vi "Single Shot Application.vi"() -> ()   [LabVIEW 2012]
doc: "This sample project is built upon the standard state machine template and shows how you could create an application that acquires, analyzes, and presents data. It includes functionality for presenting configuration dialogs, preserving settings between executions, loading and saving data, as well as exporting graph images and text files.\n\nIt is most appropriate for data that is acquired instantly as it does not allow for screen updates mid acquisition nor does it allow for continuous streaming to disk."
uses:
  controls/Acquire_Type.ctl
  controls/MDOData.ctl
  controls/MDOUI References.ctl
  controls/MDOGraph Data.ctl
  <vilib>/Utility/miscctls.llb/LVAnnotationListTypeDef.ctl
  <vilib>/Utility/miscctls.llb/LVCursorListTypeDef.ctl
  controls/MDOUser Specified Data.ctl
  controls/MDOHW Configuration.ctl
  controls/MDONew Data Behavior.ctl
  controls/Coeff.ctl
  controls/MDOState.ctl
  <vilib>/Analysis/baseanly.llb/Mean (DBL).vi
  <vilib>/Analysis/NI_AALBase.lvlib
panel:
  in  "Calibrate":bool
  out "Acquire Type":T1=enum."Continues"
  in  "Cancel":bool
  in  "Settings":bool
  in  "Snapshot":bool
  in  "Analyze":bool
  in  "Clear":bool
  in  "Stop":bool
  in  "Acquire":bool
  in  "Export":bool
  in  "Save Data":bool
  in  "Load Data":bool
  out "Mixed Signal Graph":cluster{waveform(dbl)[], waveform(dbl)[]}(graph)
  out "Status Bar":string
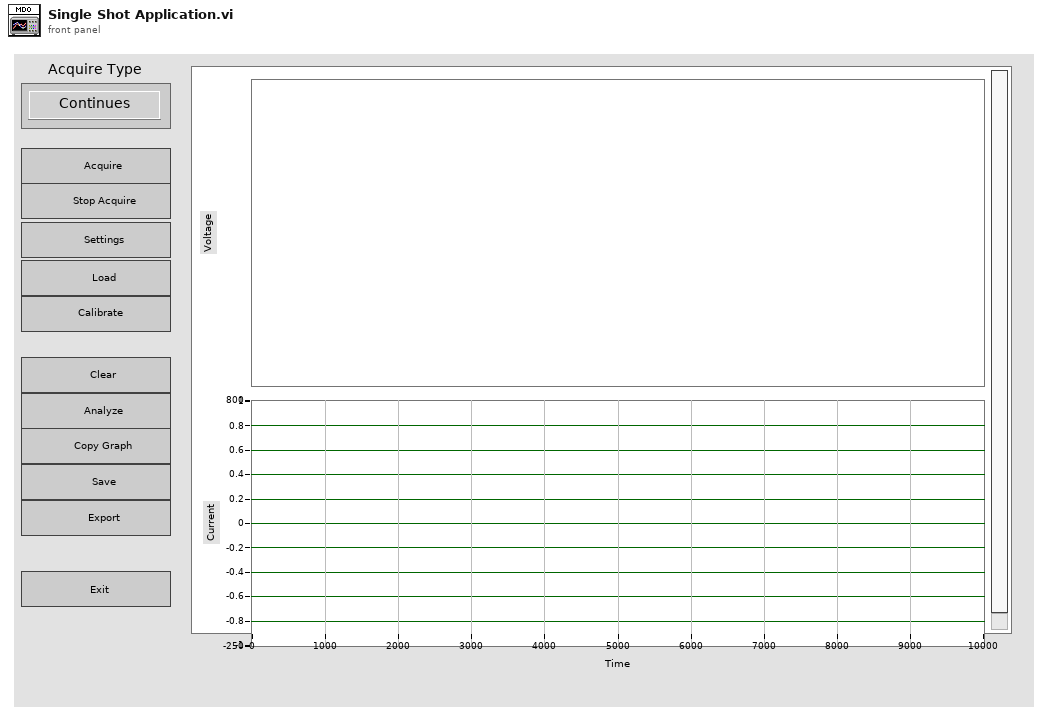
[diagram p1: front panel]
types:
  T1 = typedef "Acquire_Type.ctl" = enum16{"Triggered", "Continues"}
  T2 = typedef "MDOState.ctl" = enum16{"Wait for Event", "Initialize", "Update UI", "Configure", "Single Acquire", "Stop Contin Acquire", "Load Data", "Save Data", "Clear Data", "Export Data", "Analyze", "Copy Graph", "Calibrate", "Stop", "Run Contin Asquire", "Monitor Contin Asquire"}
  T3 = typedef "MDOData.ctl" = cluster{"UI References":T4, "Graph Data":T5, "User Specified":T8, "Coeff":T11}
  T4 = typedef "MDOUI References.ctl" = cluster{"Stop Ref":refnum<vi>, "Save Ref":refnum<vi>, "Open Ref":refnum<vi>, "Export Ref":refnum<vi>, "Acquire Ref":refnum<vi>, "Configure Ref":refnum<vi>, "Clear Ref":refnum<vi>, "Analyze Ref":refnum<vi>, "Status Ref":refnum<vi>, "Snapshot Ref":refnum<vi>, "Cancel":refnum<vi>, "Graph Ref":refnum<vi>}
  T5 = typedef "MDOGraph Data.ctl" = cluster{"Voltage Data":waveform(dbl)[], "Annotation List":T6, "Cursor List":T7, "Voltage Analysis Data":waveform(dbl)[], "Current Data":waveform(dbl)[], "Current Analysis Data":waveform(dbl)[]}
  T6 = typedef "LVAnnotationListTypeDef.ctl" = cluster{"Name":string, "Color":u32, "Style":u8, "Point Style":u8, "Name Visible":bool, "Allow Drag":bool, "Annotation Mode":u32, "Plot":i32, "Index":i32, "Position":cluster{"X":dbl, "Y":dbl}, "X Scale":u32, "Y Scale":u32, "Show Arrow":bool, "Lock Name":bool, "Plot Area":i32, "Label Offset":cluster{"X":dbl, "Y":dbl}}[]
  T7 = typedef "LVCursorListTypeDef.ctl" = cluster{"Name":string, "Color":u32, "Style":u8, "Point Style":u8, "Name Visible":bool, "Allow Drag":bool, "Cursor Mode":u32, "Plot":i32, "Index":i32, "Position":cluster{"X":dbl, "Y":dbl}, "X Scale":u32, "Y Scale":u32, "Watch Plots":i32[], "Watch All Plots":bool, "Plot Area":i32, "Label Offset":cluster{"X":dbl, "Y":dbl}}[]
  T8 = typedef "MDOUser Specified Data.ctl" = cluster{"Hardware Configuration":T9, "New Data Behavior":T10, "Acquire Type":T1, "Data_save_directory":path}
  T9 = typedef "MDOHW Configuration.ctl" = cluster{"SyncMode":u32, "Current_FIR_filter":bool}
  T10 = typedef "MDONew Data Behavior.ctl" = enum16{"Replace", "Overlay", "Append"}
  T11 = typedef "Coeff.ctl" = cluster{"Coeff_U":dbl, "Offset_U":dbl, "Coeff_I":dbl, "Offset_I":dbl}
  T12 = enum32{"invalid app kind", "Development System", "Run Time System", "Student Edition", "Embedded LabVIEW", "Evaluation", "Custom"}
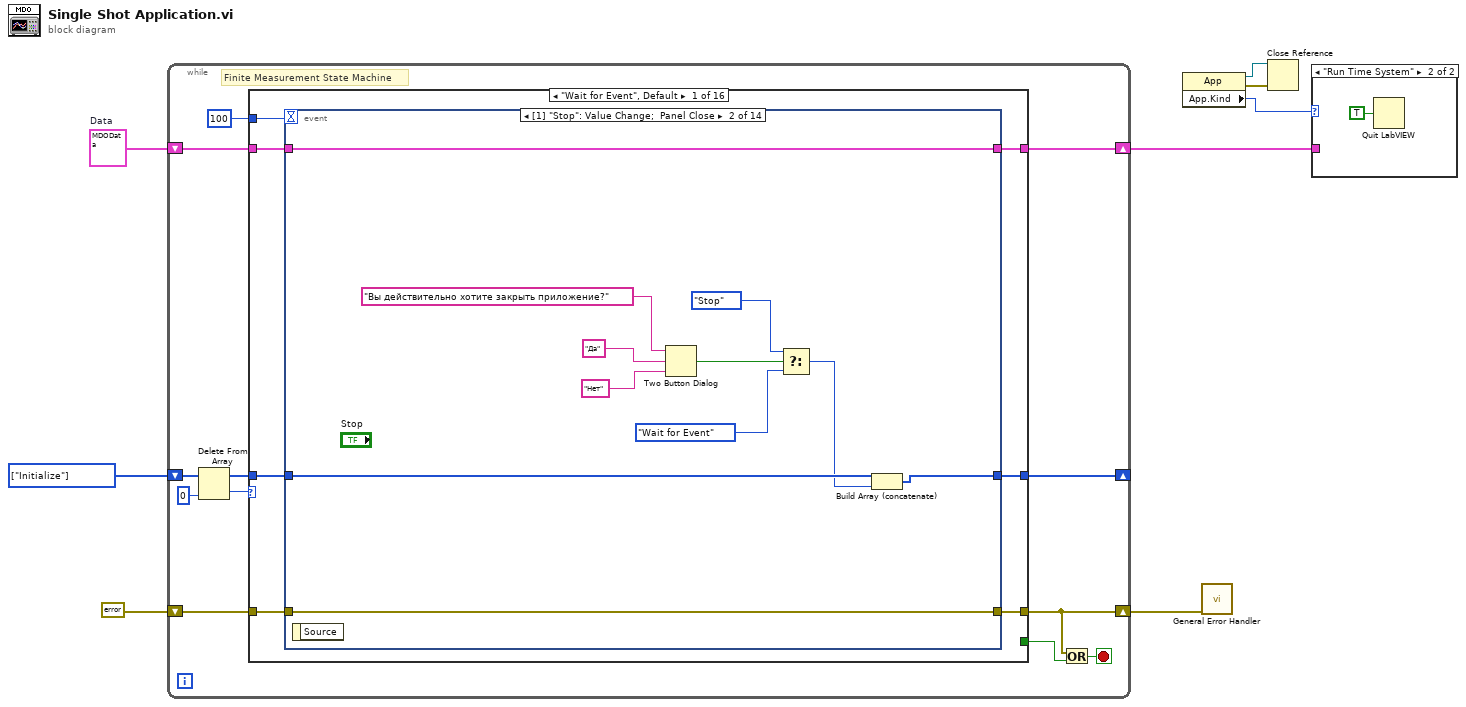
[diagram p0: block diagram]
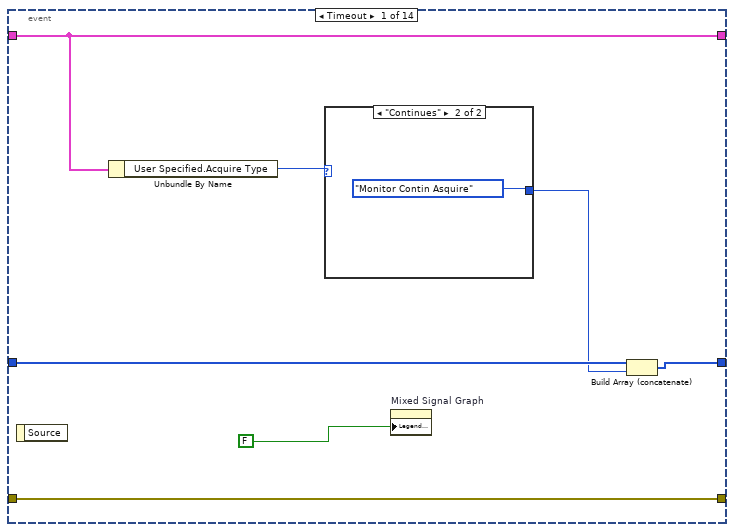
[diagram p3: hidden frame]
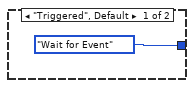
[diagram p4: hidden frame]
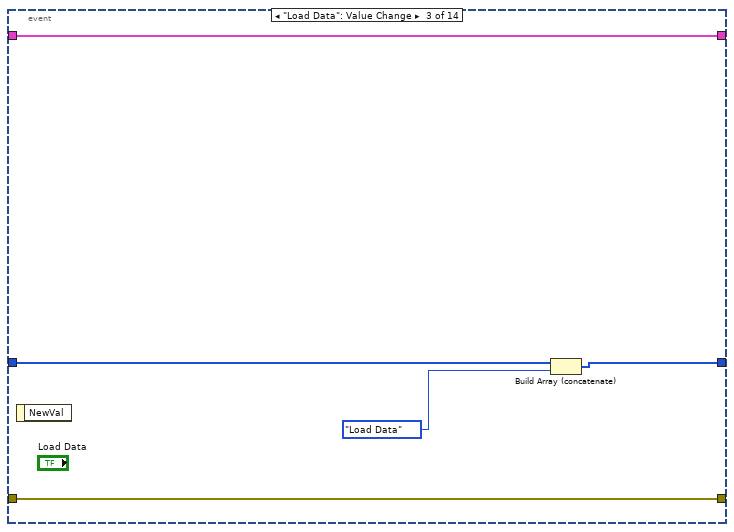
[diagram p5: hidden frame]
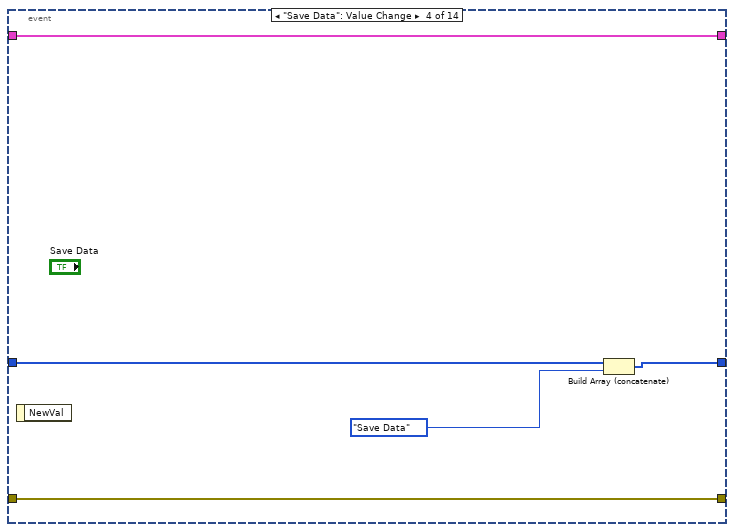
[diagram p6: hidden frame]
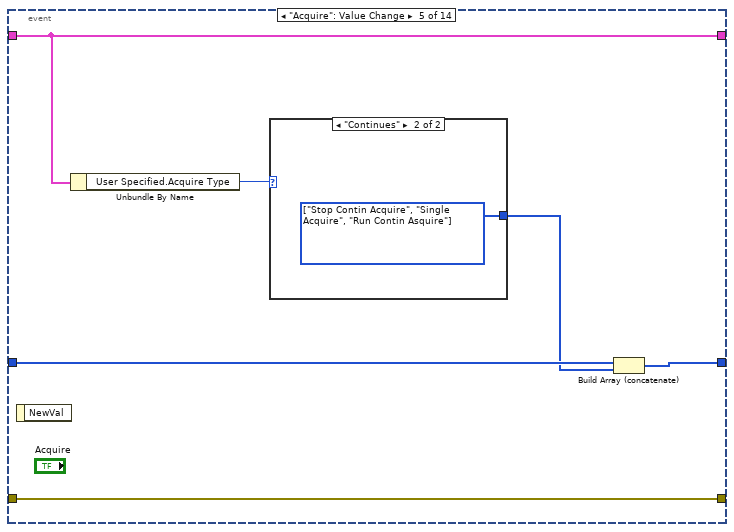
[diagram p7: hidden frame]
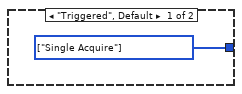
[diagram p8: hidden frame]
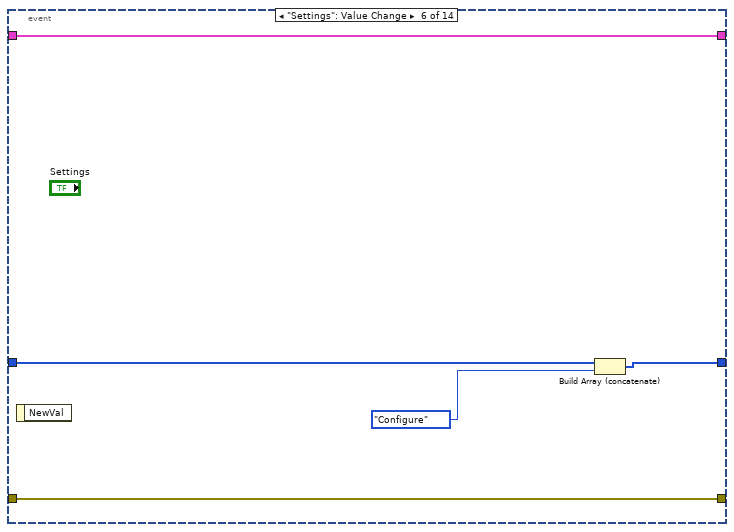
[diagram p9: hidden frame]
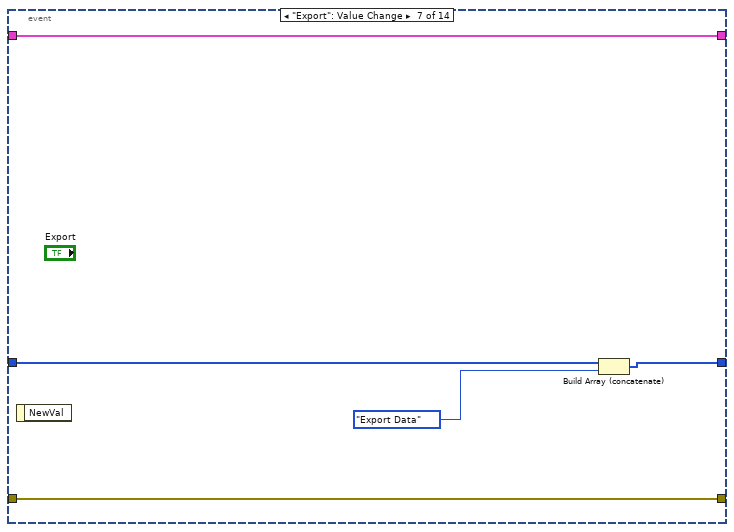
[diagram p10: hidden frame]
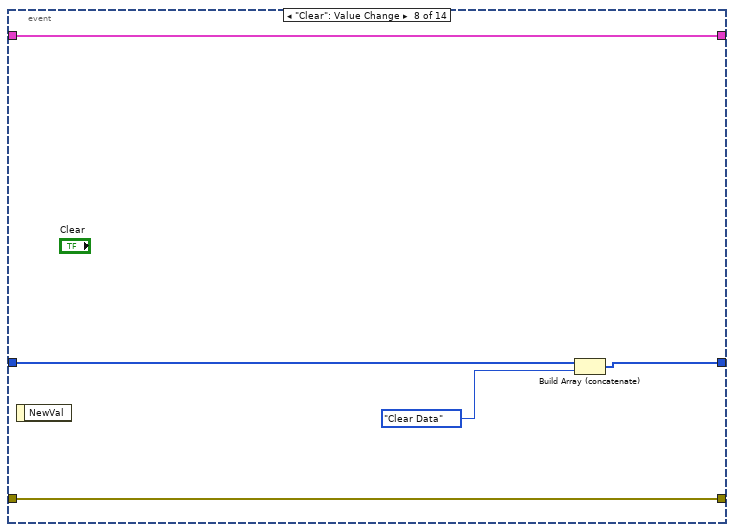
[diagram p11: hidden frame]
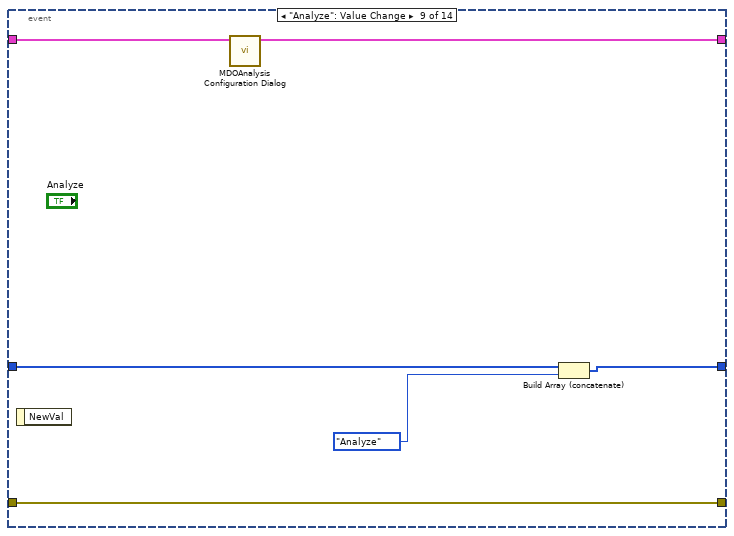
[diagram p12: hidden frame]
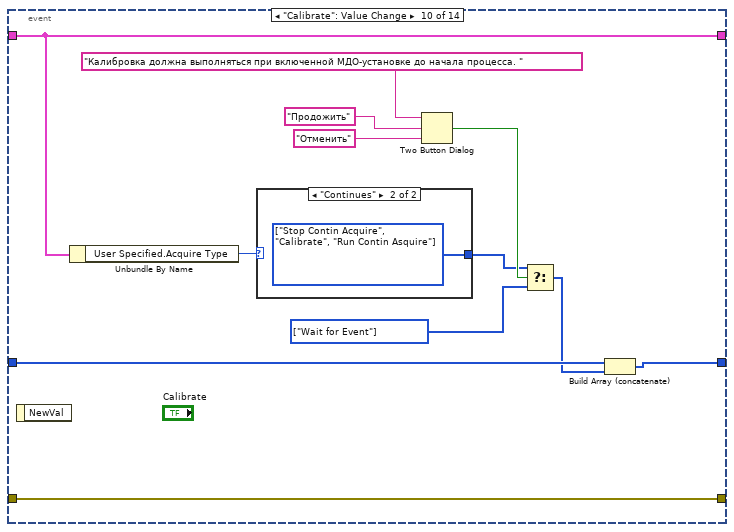
[diagram p13: hidden frame]
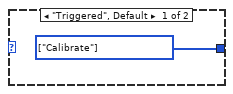
[diagram p14: hidden frame]
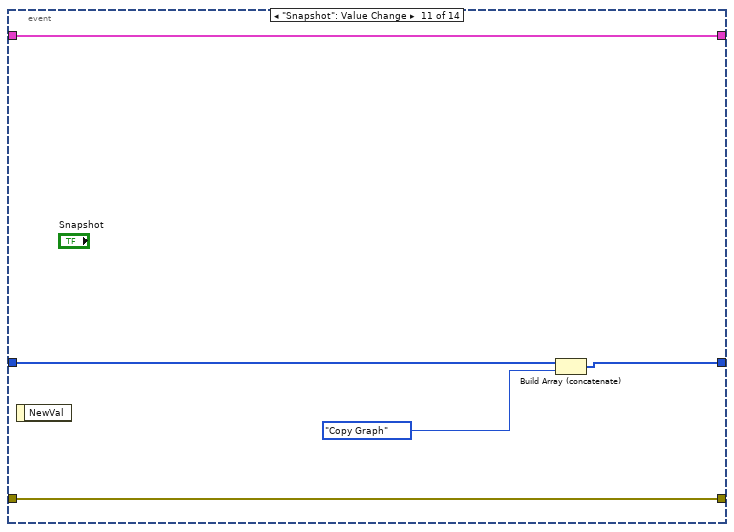
[diagram p15: hidden frame]
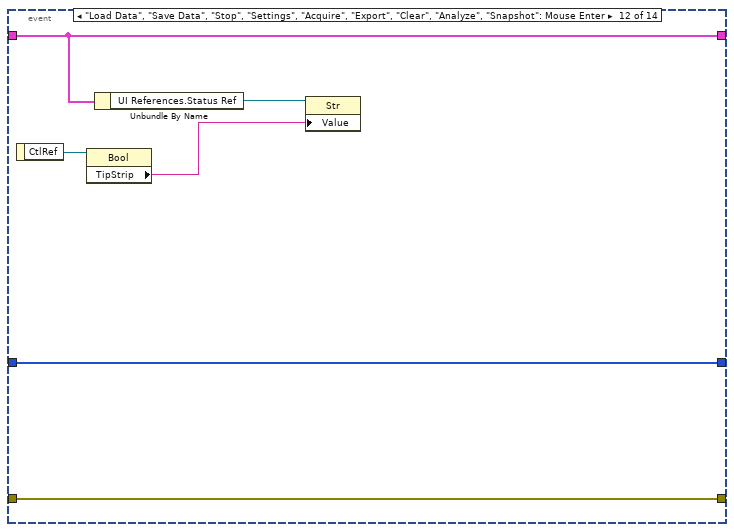
[diagram p16: hidden frame]
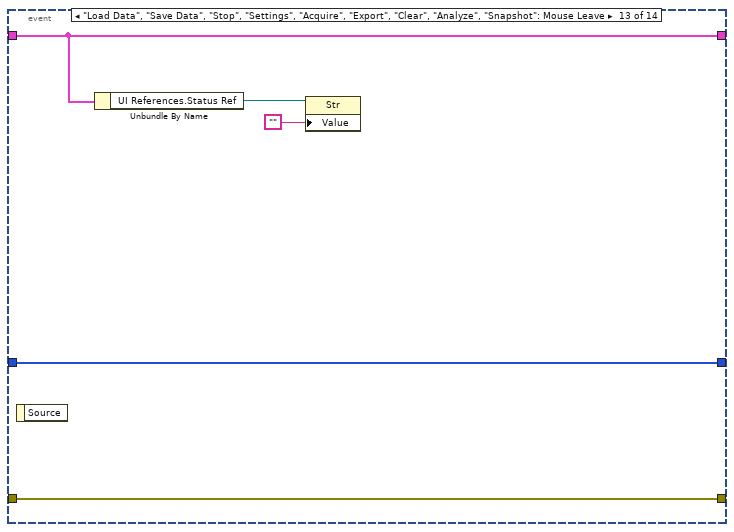
[diagram p17: hidden frame]
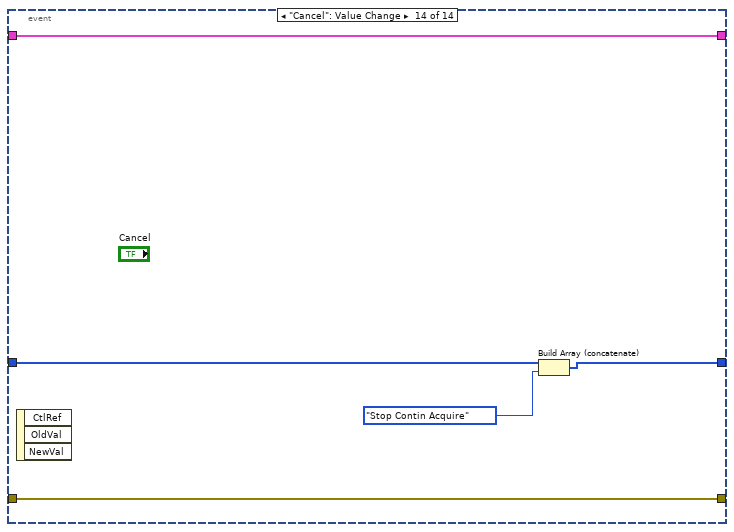
[diagram p18: hidden frame]
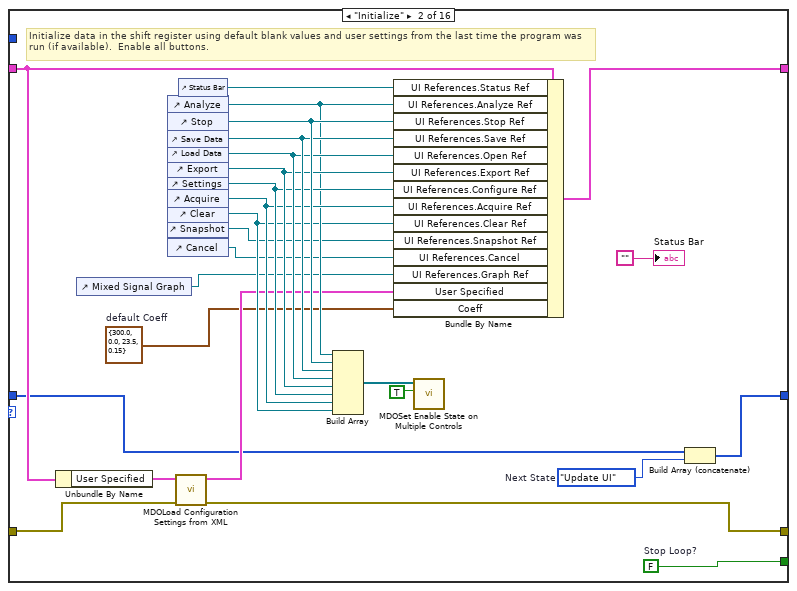
[diagram p19: hidden frame]
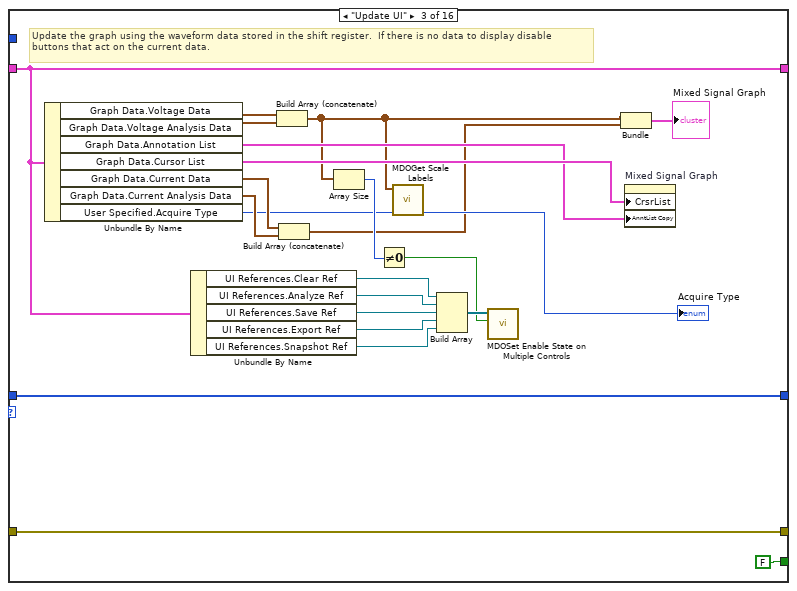
[diagram p20: hidden frame]
diagram:
  w1 = T2[] [enum."Initialize"] items=["Wait for Event", "Initialize", "Update UI", "Configure", "Single Acquire", "Stop Contin Acquire", "Load Data", "Save Data", "Clear Data", "Export Data", "Analyze", "Copy Graph", "Calibrate", "Stop", "Run Contin Asquire", "Monitor Contin Asquire"]
  w2 = T3 {"UI References"={"Stop Ref"=refnum, "Save Ref"=refnum, "Open Ref"=refnum, "Export Ref"=refnum, "Acquire Ref"=refnum, "Configure Ref"=refnum, "Clear Ref"=refnum, "Analyze Ref"=refnum, "Status Ref"=refnum, "Snapshot Ref"=refnum, "Cancel"=refnum, "Graph Ref"=refnum}, "Graph Data"={"Voltage Data"=[], "Annotation List"=[], "Cursor List"=[], "Voltage Analysis Data"=[], "Current Data"=[], "Current Analysis Data"=[]}, "User Specified"={"Hardware Configuration"={"SyncMode"=0, "Current_FIR_filter"=FALSE}, "New Data Behavior"=enum."Replace", "Acquire Type"=enum."Triggered", "Data_save_directory"=path ""}, "Coeff"={"Coeff_U"=0.0, "Offset_U"=0.0, "Coeff_I"=0.0, "Offset_I"=0.0}}  # Data
  n1 = while {
    shift-right: [w9] -> _
    shift-left: w1 -> [w14]
    shift-right: [w19] -> w3
    shift-left: w2 -> [w20]
    shift-right: [w15] -> w7
    shift-left: errorcluster {"status"=FALSE, "code"=0, "source"=""} ("error constant") -> [w18]
    stop <- w16 stop-if-true
    # "Finite Measurement State Machine"
    n2 = Delete From Array(array=w14, index=0) -> (deleted portion=w12:T2, array with subset deleted=w11:T2[])  [unwired: 1 in]
    n3 = case shown="\"Wait for Event\", Default" w12 {
      tunnel: [_ w147 FALSE ("Stop Loop?") FALSE ("Stop Loop?") FALSE ("Stop Loop?") FALSE ("Stop Loop?") FALSE ("Stop Loop?") FALSE ("Stop Loop?") FALSE ("Stop Loop?") FALSE ("Stop Loop?") FALSE ("Stop Loop?") FALSE ("Stop Loop?") FALSE ("Stop Loop?") w334 FALSE ("Stop Loop?") FALSE ("Stop Loop?")] -> w17
      tunnel: w20 -> [w27 w138 w168 w181 w195 w228 w244 w263 w276 w283 w297 w303 w310 w332 w346 w370]
      tunnel: [w26 w146 w168 w180 w194 w228 w239 w263 w275 w283 w297 w303 w309 w332 w346 w369] -> w19
      tunnel: w18 -> [w25 w125 w169 w179 w191 w226 w243 w265 w277 w286 w292 w302 w308 w329 w350 _]
      tunnel: [w24 w126 w169 w178 w192 w225 w242 w261 w277 w280 w291 w301 w308 w328 w350 w368] -> w15
      tunnel: w11 -> [w22 w124 w148 w172 w185 w221 w231 w255 w272 w278 w295 w299 w306 w327 w335 w353]
      tunnel: 100 -> [w23 _ _ _ _ _ _ _ _ _ _ _ _ _ _ _]
      tunnel: [w21 w122 w148 w170 w183 w219 w229 w255 w270 w278 w293 w299 w304 w325 w335 w351] -> w9
      frame "Wait for Event", Default {
        n4 = event shown="[1] \"Stop\": Value Change;  Panel Close" {
          selector: _ -> [_ _ _ _ _ _ _ _ _ _ _ _ _ _]
          dyn-events: _ -> [_ _ _ _ _ _ _ _ _ _ _ _ _ _]
          timeout: w23 -> [_ _ _ _ _ _ _ _ _ _ _ _ _ _]
          tunnel: w27 -> [w33 w47 w52 w57 w62 w70 w75 w80 w85 w91 w105 w109 w115 w121]
          tunnel: [w33 w47 w52 w57 w62 w70 w75 w80 w84 w91 w105 w109 w115 w121] -> w26
          tunnel: w25 -> [w34 w46 w51 w56 w63 w69 w74 w79 w86 w98 w104 w111 w116 w120]
          tunnel: [w34 w46 w51 w56 w63 w69 w74 w79 w86 w98 w104 w111 w116 w120] -> w24
          tunnel: w22 -> [w31 w45 w50 w55 w60 w68 w73 w78 w83 w93 w103 w106 w112 w119]
          tunnel: [w30 w44 w48 w53 w59 w66 w71 w76 w81 w92 w101 w106 w112 w117] -> w21
          event Timeout {
            n5 = event-data() -> ()  [unwired: 1 in, 1 out]
            n6 = Unbundle By Name(w33) -> ("User Specified.Acquire Type"=w32:T1)
            n7 = case shown="\"Continues\"" w32 {
              tunnel: [MDOState."Wait for Event" ("Next State") MDOState."Monitor Contin Asquire" ("Next State")] -> w29
              frame "Triggered", Default {
              }
              frame "Continues" {
              }
            }
            n8 = property on="Mixed Signal Graph" class="MixedGraph (strict)"("Legend Visible"=FALSE ("Boolean")) -> ()  [unwired: 2 in, 2 out]
            n9 = Build Array (concatenate)(w31, w29) -> (w30:T2[])
          }
          event "Stop": Value Change; Panel Close {
            n10 = event-data() -> ()  [unwired: 1 in, 1 out]
            n11 = Two Button Dialog(message="Вы действительно хотите закрыть приложение?", 1:"Нет" ("F button name (\"Cancel\")"), 2:"Да" ("T button name (\"OK\")")) -> (T button?=w40:bool)
            n12 = Select(t=MDOState."Stop" ("Next State"), s=w40, f=MDOState."Wait for Event" ("Next State")) -> (s? t:f=w37:T2)
            n13 = Build Array (concatenate)(w45, w37) -> (w44:T2[])
          }
          event "Load Data": Value Change {
            n14 = event-data() -> ()  [unwired: 1 in, 1 out]
            n15 = Build Array (concatenate)(w50, MDOState."Load Data" ("Next State")) -> (w48:T2[])
          }
          event "Save Data": Value Change {
            n16 = event-data() -> ()  [unwired: 1 in, 1 out]
            n17 = Build Array (concatenate)(w55, MDOState."Save Data" ("Next State")) -> (w53:T2[])
          }
          event "Acquire": Value Change {
            n18 = event-data() -> ()  [unwired: 1 in, 1 out]
            n19 = Unbundle By Name(w62) -> ("User Specified.Acquire Type"=w61:T1)
            n20 = case shown="\"Continues\"" w61 {
              tunnel: [w64 w65] -> w58
              frame "Triggered", Default {
                w64 = T2[] [enum."Single Acquire"] items=["Wait for Event", "Initialize", "Update UI", "Configure", "Single Acquire", "Stop Contin Acquire", "Load Data", "Save Data", "Clear Data", "Export Data", "Analyze", "Copy Graph", "Calibrate", "Stop", "Run Contin Asquire", "Monitor Contin Asquire"] ("array")
              }
              frame "Continues" {
                w65 = T2[] [enum."Stop Contin Acquire", enum."Single Acquire", enum."Run Contin Asquire"] items=["Wait for Event", "Initialize", "Update UI", "Configure", "Single Acquire", "Stop Contin Acquire", "Load Data", "Save Data", "Clear Data", "Export Data", "Analyze", "Copy Graph", "Calibrate", "Stop", "Run Contin Asquire", "Monitor Contin Asquire"] ("array")
              }
            }
            n21 = Build Array (concatenate)(w60, w58) -> (w59:T2[])
          }
          event "Settings": Value Change {
            n22 = event-data() -> ()  [unwired: 1 in, 1 out]
            n23 = Build Array (concatenate)(w68, MDOState."Configure" ("Next State")) -> (w66:T2[])
          }
          event "Export": Value Change {
            n24 = event-data() -> ()  [unwired: 1 in, 1 out]
            n25 = Build Array (concatenate)(w73, MDOState."Export Data" ("Next State")) -> (w71:T2[])
          }
          event "Clear": Value Change {
            n26 = event-data() -> ()  [unwired: 1 in, 1 out]
            n27 = Build Array (concatenate)(w78, MDOState."Clear Data" ("Next State")) -> (w76:T2[])
          }
          event "Analyze": Value Change {
            n28 = event-data() -> ()  [unwired: 1 in, 1 out]
            n29 = call "MDOAnalysis Configuration Dialog.vi"("Data in"=w85) -> ("Data out"=w84:T3)  [unwired: 10 in]
            n30 = Build Array (concatenate)(w83, MDOState."Analyze" ("Next State")) -> (w81:T2[])
          }
          event "Calibrate": Value Change {
            w90 = T2[] [enum."Wait for Event"] items=["Wait for Event", "Initialize", "Update UI", "Configure", "Single Acquire", "Stop Contin Acquire", "Load Data", "Save Data", "Clear Data", "Export Data", "Analyze", "Copy Graph", "Calibrate", "Stop", "Run Contin Asquire", "Monitor Contin Asquire"] ("array")
            n31 = event-data() -> ()  [unwired: 1 in, 1 out]
            n32 = Unbundle By Name(w91) -> ("User Specified.Acquire Type"=w89:T1)
            n33 = case shown="\"Continues\"" w89 {
              tunnel: [w99 w100] -> w88
              frame "Triggered", Default {
                w99 = T2[] [enum."Calibrate"] items=["Wait for Event", "Initialize", "Update UI", "Configure", "Single Acquire", "Stop Contin Acquire", "Load Data", "Save Data", "Clear Data", "Export Data", "Analyze", "Copy Graph", "Calibrate", "Stop", "Run Contin Asquire", "Monitor Contin Asquire"] ("array")
              }
              frame "Continues" {
                w100 = T2[] [enum."Stop Contin Acquire", enum."Calibrate", enum."Run Contin Asquire"] items=["Wait for Event", "Initialize", "Update UI", "Configure", "Single Acquire", "Stop Contin Acquire", "Load Data", "Save Data", "Clear Data", "Export Data", "Analyze", "Copy Graph", "Calibrate", "Stop", "Run Contin Asquire", "Monitor Contin Asquire"] ("array")
              }
            }
            n34 = Two Button Dialog(message="Калибровка должна выполняться при включенной МДО-установке до начала процесса. ", 1:"Отменить" ("F button name (\"Cancel\")"), 2:"Продожить" ("T button name (\"OK\")")) -> (T button?=w94:bool)
            n35 = Select(t=w88, s=w94, f=w90) -> (s? t:f=w87:T2[])
            n36 = Build Array (concatenate)(w93, w87) -> (w92:T2[])
          }
          event "Snapshot": Value Change {
            n37 = event-data() -> ()  [unwired: 1 in, 1 out]
            n38 = Build Array (concatenate)(w103, MDOState."Copy Graph" ("Next State")) -> (w101:T2[])
          }
          event "Load Data", "Save Data", "Stop", "Settings", "Acquire", "Export", "Clear", "Analyze", "Snapshot": Mouse Enter {
            n39 = event-data() -> ("CtlRef"=w110:refnum<vi>)  [unwired: 1 in]
            n40 = property class="Bool"(reference=w110) -> ("TipStrip"=w107:string)  [unwired: 1 in, 2 out]
            n41 = Unbundle By Name(w109) -> ("UI References.Status Ref"=w108:refnum<vi>)
            n42 = property class="Str"(reference=w108, "Value"=w107) -> ()  [unwired: 1 in, 2 out]
          }
          event "Load Data", "Save Data", "Stop", "Settings", "Acquire", "Export", "Clear", "Analyze", "Snapshot": Mouse Leave {
            n43 = event-data() -> ()  [unwired: 1 in, 1 out]
            n44 = Unbundle By Name(w115) -> ("UI References.Status Ref"=w114:refnum<vi>)
            n45 = property class="Str"(reference=w114, "Value"="") -> ()  [unwired: 1 in, 2 out]
          }
          event "Cancel": Value Change {
            n46 = event-data() -> ()  [unwired: 1 in, 3 out]
            n47 = Build Array (concatenate)(w119, MDOState."Stop Contin Acquire" ("Initial State")) -> (w117:T2[])
          }
        }
      }
      frame "Initialize" {
        w127 = T11 {"Coeff_U"=300.0, "Offset_U"=0.0, "Coeff_I"=23.5, "Offset_I"=0.15}  # default Coeff
        w147 = FALSE  # Stop Loop?
        w123 = MDOState."Update UI"  # Next State
        # "Initialize data in the shift register using default blank values and user settings from the last time the program was run (if available).  Enable all buttons."
        n48 = Unbundle By Name(w138) -> ("User Specified"=w137:T8)
        n49 = control-ref of="Mixed Signal Graph"() -> (w128:refnum<vi>)
        n50 = control-ref of="Analyze"() -> (w136:refnum<vi>)
        n51 = control-ref of="Stop"() -> (w145:refnum<vi>)
        n52 = control-ref of="Save Data"() -> (w144:refnum<vi>)
        n53 = control-ref of="Load Data"() -> (w143:refnum<vi>)
        n54 = control-ref of="Export"() -> (w142:refnum<vi>)
        n55 = control-ref of="Settings"() -> (w141:refnum<vi>)
        n56 = control-ref of="Acquire"() -> (w140:refnum<vi>)
        n57 = control-ref of="Clear"() -> (w134:refnum<vi>)
        n58 = control-ref of="Snapshot"() -> (w131:refnum<vi>)
        n59 = control-ref of="Cancel"() -> (w129:refnum<vi>)
        n60 = call "MDOLoad Configuration Settings from XML.vi"("error in (no error)"=w125, "User Configuration in"=w137) -> ("error out"=w126:errorcluster, "User Configuration out"=w130:T8)  [unwired: 8 in]
        n61 = control-ref of="Status Bar"() -> (w135:refnum<vi>)
        n62 = Build Array(w136, w145, w144, w143, w142, w141, w140, w134) -> (w139:refnum<vi>[])
        n63 = Bundle By Name(cluster=w138, "UI References.Status Ref"=w135, "UI References.Analyze Ref"=w136, "UI References.Stop Ref"=w145, "UI References.Save Ref"=w144, "UI References.Open Ref"=w143, "UI References.Export Ref"=w142, "UI References.Configure Ref"=w141, "UI References.Acquire Ref"=w140, "UI References.Clear Ref"=w134, "UI References.Snapshot Ref"=w131, "UI References.Cancel"=w129, "UI References.Graph Ref"=w128, "User Specified"=w130, "Coeff"=w127) -> (w146:T3)
        n64 = call "MDOSet Enable State on Multiple Controls.vi"("Enable?"=TRUE, "Controls"=w139) -> ()  [unwired: 10 in]
        n65 = Build Array (concatenate)(w124, w123) -> (w122:T2[])
        "Status Bar" <- "" ("Status Bar")
      }
      frame "Update UI" {
        # "Update the graph using the waveform data stored in the shift register.  If there is no data to display disable buttons that act on the current data."
        n66 = Unbundle By Name(w168) -> ("Graph Data.Voltage Data"=w165:waveform(dbl)[], "Graph Data.Voltage Analysis Data"=w159:waveform(dbl)[], "Graph Data.Annotation List"=w153:T6, "Graph Data.Cursor List"=w154:T7, "Graph Data.Current Data"=w158:waveform(dbl)[], "Graph Data.Current Analysis Data"=w157:waveform(dbl)[], "User Specified.Acquire Type"=→"Acquire Type":T1)
        n67 = Unbundle By Name(w168) -> ("UI References.Clear Ref"=w163:refnum<vi>, "UI References.Analyze Ref"=w162:refnum<vi>, "UI References.Save Ref"=w167:refnum<vi>, "UI References.Export Ref"=w160:refnum<vi>, "UI References.Snapshot Ref"=w161:refnum<vi>)
        n68 = Build Array (concatenate)(w165, w159) -> (w152:waveform(dbl)[])
        n69 = Build Array (concatenate)(w158, w157) -> (w151:waveform(dbl)[])
        n70 = Array Size(array=w152) -> (size(s)=w156:i32)
        n71 = Not Equal To 0?(x=w156) -> (x != 0?=w164:bool)
        n72 = call "MDOGet Scale Labels.vi"("Array of Waveforms"=w152) -> ()  [unwired: 9 in, 2 out]
        n73 = Build Array(w163, w162, w167, w160, w161) -> (w166:refnum<vi>[])
        n74 = call "MDOSet Enable State on Multiple Controls.vi"("Enable?"=w164, "Controls"=w166) -> ()  [unwired: 10 in]
        n75 = Bundle(w152, w151) -> (→"Mixed Signal Graph":cluster{waveform(dbl)[], waveform(dbl)[]})  [unwired: 1 in]
        n76 = property on="Mixed Signal Graph" class="MixedGraph (strict)"("CrsrList"=w154, "AnntList Copy"=w153) -> ()  [unwired: 2 in, 2 out]
      }
      frame "Configure" {
        # "Spawns a dialog that allows the user to set any user configurable settings."
        n77 = Unbundle By Name(w181) -> ("User Specified"=w174:T8)
        n78 = call "MDOSettings Dialog.vi"("error in (no error)"=w179, "Configuration in"=w174) -> ("error out"=w178:errorcluster, "UI Refresh Needed?"=w177:bool, "Configuration out"=w173:T8)  [unwired: 7 in]
        n79 = Bundle By Name(cluster=w181, "User Specified"=w173) -> (w180:T3)
        n80 = Select(t=MDOState."Update UI" ("Next State if true"), s=w177, f=MDOState."Wait for Event" ("Next State if false")) -> (s? t:f=w171:T2)
        n81 = Build Array (concatenate)(w172, w171) -> (w170:T2[])
      }
      frame "Single Acquire" {
        # "Uses the current hardware configuration to acquire a new data set and stores it in the state data."
        n82 = Unbundle By Name(w195) -> ("UI References.Status Ref"=w193:refnum<vi>, "User Specified.Hardware Configuration"=w187:T9, "Coeff"=w186:T11)
        n83 = disable-structure shown="Enabled" {
          disable-tunnel: w191 -> [w201 w208]
          disable-tunnel: [w198 w207] -> w190
          disable-tunnel: [w200 w206] -> w189
          disable-tunnel: [w199 w205] -> w188
          disable-tunnel: w187 -> [w203 w204]
          disable-tunnel: w186 -> [w202 _]
          frame Enabled {
            n84 = call "MDOAcquire Data from х502.vi"("error in (no error)"=w201, "Coeff"=w202, "Hardware Configuration"=w203) -> ("error out"=w198:errorcluster, "Ток"=w199:dbl[], "Напряжение"=w200:dbl[])  [unwired: 6 in]
          }
          frame Disabled {
            n85 = call "MDOAcquire Data from Hardware.vi"("error in (no error)"=w208, "Hardware Configuration"=w204) -> ("error out"=w207:errorcluster, "Current"=w205:dbl[], "Voltage"=w206:dbl[])  [unwired: 6 in]
          }
        }
        n86 = case shown="No Error" w190 {
          selector: w190 -> [w213 w217]
          tunnel: w195 -> [w212 w218]
          tunnel: [w215 w218] -> w194
          tunnel: [w214 _] -> w192
          tunnel: ["Data acquired." ("Data acquired") "Data not acquired." ("Data not acquired")] -> w196
          tunnel: w189 -> [w210 _]
          tunnel: w188 -> [w209 _]
          frame No Error {
            n87 = call "MDOIncorporate New Data.vi"("error in (no error)"=w213, "New Current Data"=w209, "New Voltage Data"=w210, "Data in"=w212) -> ("error out"=w214:errorcluster, "Data out"=w215:T3)  [unwired: 6 in]
          }
          frame Error {
            n88 = call <vilib>:"Simple Error Handler.vi"("error in (no error)"=w217) -> ()  [unwired: 4 in, 5 out]
          }
        }
        n89 = Build Array (concatenate)(w185, MDOState."Update UI" ("Next State")) -> (w183:T2[])
        n90 = property class="Str"(reference=w193, "Value"=w196) -> ()  [unwired: 1 in, 2 out]
      }
      frame "Stop Contin Acquire" {
        n91 = vi-ref "MDOAcquire Data from х502 streaming.vi"() -> (w227:refnum<vi>)
        n92 = call "Write_control.vi"("error in (no error)"=w226, "data"=TRUE, "control_label"="stop", "VI ref in"=w227) -> ("error out"=w225:errorcluster)  [unwired: 6 in, 1 out]
        n93 = Build Array (concatenate)(w221, MDOState."Update UI" ("(Value Not Used)")) -> (w219:T2[])
      }
      frame "Load Data" {
        # "Loads data from an LVM file and incorporates it with the existing data according to the user's preference."
        n94 = call "MDOLoad Data.vi"("error in (no error)"=w243) -> ("error out"=w241:errorcluster, "New Graph Data"=w237:waveform(dbl)[])  [unwired: 9 in]
        n95 = Index Array(array=w237, index #1=0 ("index"), index #2=1 ("index")) -> (element #1=w234:waveform(dbl), element #2=w233:waveform(dbl))
        n96 = case shown="No Error" w241 {
          selector: w241 -> [w249 w253]
          tunnel: w244 -> [w248 w254]
          tunnel: [w251 w254] -> w239
          tunnel: [w250 _] -> w242
          tunnel: ["Data loaded." ("Data loaded") "Data not loaded." ("Data not loaded")] -> w240
          tunnel: w234 -> [w246 _]
          tunnel: w233 -> [w245 _]
          frame No Error {
            n97 = call "MDOIncorporate New Data.vi"("error in (no error)"=w249, "New Current Data"=w245, "New Voltage Data"=w246, "Data in"=w248) -> ("error out"=w250:errorcluster, "Data out"=w251:T3)  [unwired: 6 in]
          }
          frame Error {
            n98 = call <vilib>:"Simple Error Handler.vi"("error in (no error)"=w253) -> ()  [unwired: 4 in, 5 out]
          }
        }
        n99 = Unbundle By Name(w239) -> ("UI References.Status Ref"=w238:refnum<vi>)
        n100 = property class="Str"(reference=w238, "Value"=w240) -> ()  [unwired: 1 in, 2 out]
        n101 = Build Array (concatenate)(w231, MDOState."Update UI" ("(Value Not Used)")) -> (w229:T2[])
      }
      frame "Save Data" {
        # "Saves the existing measurement data to an LVM file."
        n102 = Unbundle By Name(w263) -> ("User Specified.Data_save_directory"=w257:path, "UI References.Status Ref"=w262:refnum<vi>, "Graph Data.Voltage Data"=w259:waveform(dbl)[], "Graph Data.Current Data"=w258:waveform(dbl)[])
        n103 = call "MDOSave Data.vi"("Data_save_directory"=w257, "error in (no error)"=w265, "Current Data"=w258, "Voltage Data"=w259) -> ("error out"=w264:errorcluster)  [unwired: 7 in]
        n104 = case shown="No Error" w264 {
          selector: w264 -> [w266 w269]
          tunnel: ["Data saved." ("Data saved") "Data not saved." ("Data not saved")] -> w260
          tunnel: [w266 _] -> w261
          frame No Error {
          }
          frame Error {
            n105 = call <vilib>:"Simple Error Handler.vi"("error in (no error)"=w269) -> ()  [unwired: 4 in, 5 out]
          }
        }
        n106 = property class="Str"(reference=w262, "Value"=w260) -> ()  [unwired: 1 in, 2 out]
      }
      frame "Clear Data" {
        w274 = T5 {"Voltage Data"=[], "Annotation List"=[], "Cursor List"=[], "Voltage Analysis Data"=[], "Current Data"=[], "Current Analysis Data"=[]}  # Graph
        # "Clears the data currently in the graph."
        n107 = Bundle By Name(cluster=w276, "Graph Data"=w274) -> (w275:T3)
        n108 = Build Array (concatenate)(w272, MDOState."Update UI" ("(Value Not Used)")) -> (w270:T2[])
      }
      frame "Export Data" {
        # "Exports the currently loaded measurement and analysis data to a text file that can be imported into a spreadsheet or other application."
        n109 = Unbundle By Name(w283) -> ("UI References.Status Ref"=w281:refnum<vi>, "Graph Data"=w282:T5)
        n110 = call "MDOExport Data.vi"("error in (no error)"=w286, "Graph Data"=w282) -> ("error out"=w284:errorcluster)  [unwired: 9 in]
        n111 = case shown="No Error" w284 {
          selector: w284 -> [w287 w290]
          tunnel: ["Data exported." ("Data exported") "Data not exported." ("Data not exported")] -> w285
          tunnel: [w287 _] -> w280
          frame No Error {
          }
          frame Error {
            n112 = call <vilib>:"Simple Error Handler.vi"("error in (no error)"=w290) -> ()  [unwired: 4 in, 5 out]
          }
        }
        n113 = property class="Str"(reference=w281, "Value"=w285) -> ()  [unwired: 1 in, 2 out]
      }
      frame "Analyze" {
        # "Code Recommended - Add your own signal analysis here."
        # "Analyzes the measurement data."
        n114 = Unbundle By Name(w297) -> ("Graph Data"=w298:T5)
        n115 = call "MDOStatistical Analysis.vi"("error in (no error)"=w292, "Graph Data In"=w298) -> ("error out"=w291:errorcluster)  [unwired: 7 in, 1 out]
        n116 = Build Array (concatenate)(w295, MDOState."Update UI" ("(Value Not Used)")) -> (w293:T2[])
      }
      frame "Copy Graph" {
        # "Places an image of the graph on the clipboard for pasting into reports or emails."
        n117 = call "MDOCopy Graph to Clipboard.vi"("error in (no error)"=w302, "Graph Data"=w303) -> ("error out"=w301:errorcluster)  [unwired: 9 in]
      }
      frame "Calibrate" {
        n118 = in-place {
          w317 = u32 0 items=["INTERNAL"=0, "EXTERNAL_MASTER"=1, "DI_SYN1_RISE"=2, "DI_SYN1_FALL"=3, "DI_SYN2_RISE"=6, "DI_SYN2_FALL"=7] ("SyncMode")
          # "сложение здесь потому-что канал\nтока инвертирован в subVI сора данных"
          n119 = in-place-cluster #1(w310) -> ("Coeff"=w314:T11, "User Specified.Hardware Configuration"=w316:T9)
          n120 = Bundle By Name(cluster=w316, "SyncMode"=w317) -> (w315:T9)
          n121 = call "MDOAcquire Data from х502.vi"("Coeff"=w314, "Hardware Configuration"=w315) -> ("error out"=w313:errorcluster, "Ток"=w311:dbl[], "Напряжение"=w312:dbl[])  [unwired: 7 in]
          n122 = Unbundle By Name(w314) -> ("Offset_U"=w323:dbl, "Offset_I"=w322:dbl)
          n123 = call-poly <vilib>:"Mean.vi"("X"=w311) -> ("mean"=w320:dbl)  [unwired: 1 out]
          n124 = call-poly <vilib>:"Mean.vi"("X"=w312) -> ("mean"=w321:dbl)  [unwired: 1 out]
          n125 = Subtract(x=w323, y=w321) -> (x-y=w319:dbl)
          n126 = Add(x=w322, y=w320) -> (x+y=w318:dbl)
          n127 = call <vilib>:"Simple Error Handler.vi"("error in (no error)"=w313) -> ()  [unwired: 4 in, 5 out]
          n128 = Bundle By Name(cluster=w314, "Offset_U"=w319, "Offset_I"=w318) -> (w324:T11)
          n129 = in-place-cluster #1("Coeff"=w324, "User Specified.Hardware Configuration"=w316) -> (w309:T3)
        }
        n130 = Build Array (concatenate)(w306, MDOState."Update UI" ("(Value Not Used)")) -> (w304:T2[])
      }
      frame "Stop" {
        w334 = TRUE  # Stop Loop?
        # "Saves the users settings to an XML file and stops execution."
        n131 = Unbundle By Name(w332) -> ("UI References.Status Ref"=w330:refnum<vi>, "User Specified"=w333:T8)
        n132 = call "MDOSave Configuration Settings to XML.vi"("error in (no error)"=w329, "User Configuration"=w333) -> ("error out"=w328:errorcluster)  [unwired: 9 in]
        n133 = property class="Str"(reference=w330, "Value"="Stopped." ("Stopped")) -> ()  [unwired: 1 in, 2 out]
        n134 = Build Array (concatenate)(w327, MDOState."Stop" ("(Value Not Used)")) -> (w325:T2[])
      }
      frame "Run Contin Asquire" {
        w349 = FALSE ("Wait Until Done")
        n135 = Unbundle By Name(w346) -> ("User Specified.Hardware Configuration"=w337:T9, "Coeff"=w338:T11)
        n136 = vi-ref "MDOAcquire Data from х502 streaming.vi"() -> (w345:refnum<vi>)
        n137 = call "Write_control.vi"("data"=w338, "control_label"="Coeff", "VI ref in"=w345) -> ("error out"=w343:errorcluster, "ref out"=w341:refnum<vi>)  [unwired: 7 in]
        n138 = call "Write_control.vi"("error in (no error)"=w343, "data"=w337, "control_label"="Hardware Configuration", "VI ref in"=w341) -> ("error out"=w342:errorcluster, "ref out"=w340:refnum<vi>)  [unwired: 6 in]
        n139 = invoke class="VI" method="Run VI"(reference=w340, error in=w342, "Wait until done"=w349, "Auto Dispose Ref"=w349) -> (reference out=w347:refnum<vi>, error out=w348:errorcluster)  [unwired: 1 in, 3 out]
        n140 = Close Reference(reference=w347, error in (no error)=w348) -> ()  [unwired: 1 out]
      }
      frame "Monitor Contin Asquire" {
        w357 = dbl[] [] ("Напряжение")
        n141 = vi-ref "MDOAcquire Data from х502 streaming.vi"() -> (w367:refnum<vi>)
        n142 = call "Read_indicator.vi"("Idicator_label"="Напряжение", "VI Refnum"=w367) -> ("error out"=w363:errorcluster, "data"=w362:variant, "ref out"=w365:refnum<vi>)  [unwired: 7 in]
        n143 = call "Read_indicator.vi"("error in"=w363, "Idicator_label"="Ток", "VI Refnum"=w365) -> ("error out"=w360:errorcluster, "data"=w361:variant)  [unwired: 6 in, 1 out]
        n144 = Variant To Data(error in=w360, type=w357, Variant=w362) -> (data=w356:dbl[], error out=w359:errorcluster)
        n145 = Variant To Data(error in=w359, type=w357, Variant=w361) -> (data=w355:dbl[], error out=w358:errorcluster)
        n146 = Build Array (concatenate)(w353, MDOState."Update UI" ("(Value Not Used)")) -> (w351:T2[])
        n147 = call "MDOIncorporate New Data.vi"("error in (no error)"=w358, "New Current Data"=w355, "New Voltage Data"=w356, "Data in"=w370) -> ("error out"=w368:errorcluster, "Data out"=w369:T3)  [unwired: 6 in]
      }
    }
    n148 = Or(x=w15, y=w17) -> (x .or. y?=w16:bool)
  }
  n149 = property class="App"() -> (reference out=w6:refnum<vi>, error out=w5:errorcluster, "App.Kind"=w4:T12)  [unwired: 2 in]
  n150 = call <vilib>:"General Error Handler.vi"("error in (no error)"=w7) -> ()  [unwired: 10 in, 5 out]
  n151 = Close Reference(reference=w6, error in (no error)=w5) -> ()  [unwired: 1 out]
  n152 = case shown="\"Run Time System\"" w4 {
    tunnel: w3 -> [_ _]
    frame "Development System", Default {
    }
    frame "Run Time System" {
      n153 = Quit LabVIEW(quit? (T)=TRUE) -> ()
    }
  }
